vi "UUT - Receive QAM Data.vi"(8 "error in (no error)":errorcluster, 11 "VISA resource name":refnum<visa-resource-name>) -> (0 "error out":errorcluster, 2 "QAM Data Out":cluster{dbl[], dbl[]}, 3 "VISA resource name out":refnum<visa-resource-name>)   [LabVIEW 2011]
uses:
  Antenna Simulation States.ctl
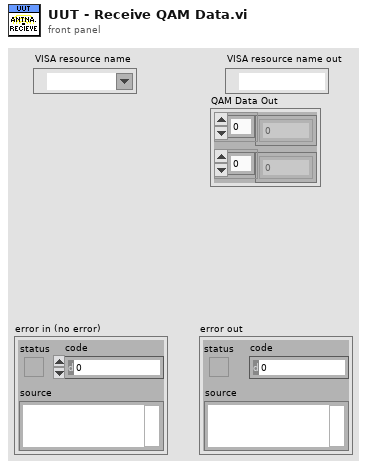
[diagram p1: front panel]
types:
  T1 = typedef "Antenna Simulation States.ctl" = enum16{"Simulate Transmit Antenna QAM Data", "Simulate Receive Antenna QAM Data"}
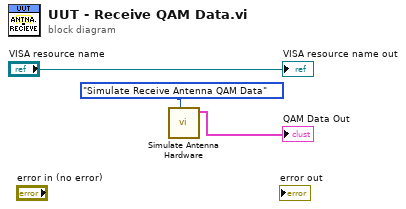
[diagram p0: block diagram]
diagram:
  n1 = call "Simulate Antenna Hardware.vi"("Command to Simulate"=Antenna_Simulation_States."Simulate Receive Antenna QAM Data") -> ("QAM Data Out"=→"QAM Data Out":cluster{dbl[], dbl[]})  [unwired: 9 in, 1 out]
  "VISA resource name out" <- "VISA resource name"
